vi "Sequence Get by Key.vi"(8 "error in (no error)":errorcluster, 10 "ixSequence":i32, 11 "Connection Refnum":T1) -> (0 "error out":errorcluster, 2 "Sequence Record":T2, 3 "Connection Refnum":T1, 4 "Data Present":bool)   [LabVIEW 2011]
uses:
  Sequence Record.ctl
  SI.LIB/ODBC/SQL Controls/Connection Refnum.ctl
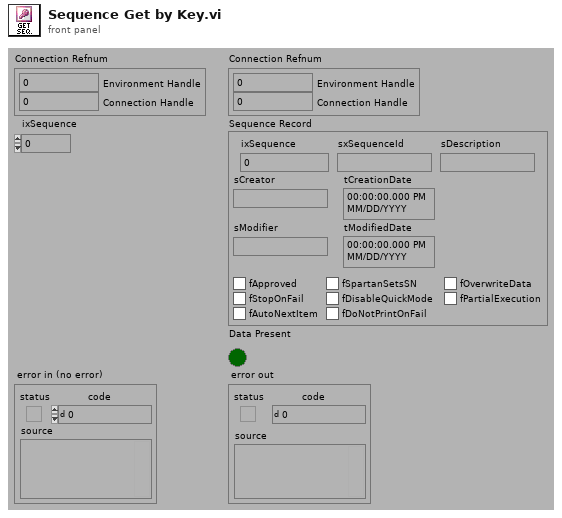
[diagram p1: front panel]
types:
  T1 = typedef "Connection Refnum.ctl" = cluster{"Environment Handle":i32, "Connection Handle":i32}
  T2 = typedef "Sequence Record.ctl" = cluster{"ixSequence":i32, "sxSequenceId":string, "sDescription":string, "sCreator":string, "tCreationDate":timestamp, "sModifier":string, "tModifiedDate":timestamp, "fApproved":bool, "fSpartanSetsSN":bool, "fOverwriteData":bool, "fStopOnFail":bool, "fDisableQuickMode":bool, "fPartialExecution":bool, "fAutoNextItem":bool, "fDoNotPrintOnFail":bool}
  T3 = typedef "Statement Refnum.ctl" = cluster{"Statement Handle":i32, "Parameter Number":u16}
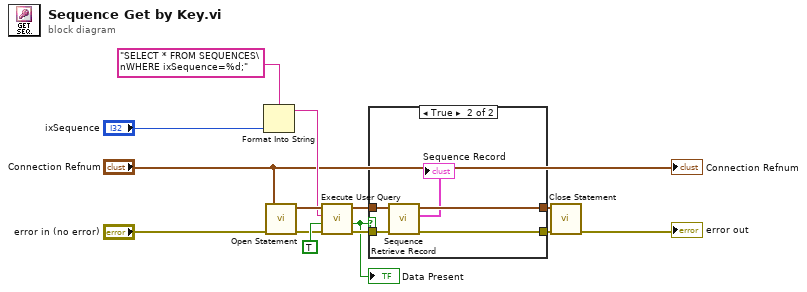
[diagram p0: block diagram]
diagram:
  n1 = Format Into String(format string="SELECT * FROM SEQUENCES\nWHERE ixSequence=%d;" ("User Query"), "ixSequence") -> (resulting string=w6:string)  [unwired: 2 in, 1 out]
  n2 = call "Open Statement.vi"("error in (no error)"="error in (no error)", "Connection Refnum"="Connection Refnum") -> ("error out"=w7:errorcluster, "Statement Refnum"=w8:T3)  [unwired: 4 out]
  n3 = call "Execute User Query.vi"("error in (no error)"=w7, "Return Data? (f)"=TRUE, "User Query"=w6, "Statement Refnum"=w8) -> ("error out"=w14:errorcluster, "Data Present?"=w5:bool, "Statement Refnum"=w13:T3)  [unwired: 1 out]
  "Data Present" <- w5
  n4 = case shown="True" w5 {
    tunnel: w14 -> [w15 w20]
    tunnel: w13 -> [w16 w21]
    tunnel: [w15 w18] -> w10
    tunnel: [w16 w19] -> w11
    frame False {
    }
    frame True {
      n5 = call "Sequence Retrieve Record.vi"("error in (no error)"=w20, "Statement Refnum"=w21) -> ("error out"=w18:errorcluster, "Sequence Record"=→"Sequence Record":T2, "Statement Refnum"=w19:T3)  [unwired: 7 out]
    }
  }
  n6 = call "Close Statement.vi"("error in (no error)"=w10, "Statement Refnum"=w11) -> ("error out"=→"error out":errorcluster)  [unwired: 5 out]
  "Connection Refnum" <- "Connection Refnum"
